vi "Dequeue Events.vi"(8 "error in (no error)":errorcluster, 10 "timeout in ms (-1)":i32, 11 "Queue in":refnum<queue>) -> (0 "error out":errorcluster, 2 "timed out?":bool, 3 "Actor Events":T1)   [LabVIEW 2017, in "Command Handler.lvlib" / "Command Handler.lvclass"]
uses:
  Command Handler.lvclass
  Type Defs/Event Cluster.ctl
  Command Parent/Command.lvclass
  Type Defs/Command Handler Data.ctl
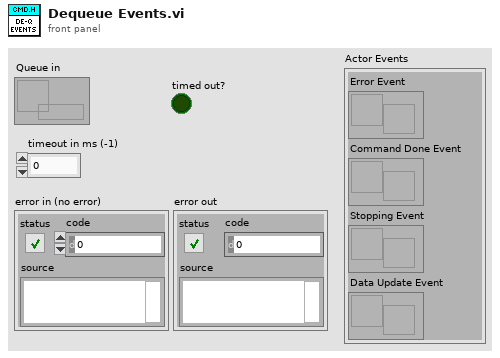
[diagram p1: front panel]
types:
  T1 = typedef "Command Handler.lvlib/Command Handler.lvclass/Event Cluster.ctl" = cluster{"Error Event":refnum<user-event>, "Command Done Event":refnum<user-event>, "Stopping Event":refnum<user-event>, "Data Update Event":refnum<user-event>}
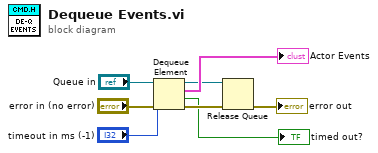
[diagram p0: block diagram]
diagram:
  n1 = Dequeue Element(queue="Queue in", timeout in ms (-1)="timeout in ms (-1)", error in (no error)="error in (no error)") -> (queue out=w6:refnum<queue>, element=→"Actor Events":T1, timed out?=→"timed out?":bool, error out=w5:errorcluster)
  n2 = Release Queue(queue=w6, error in (no error)=w5) -> (error out=→"error out":errorcluster)  [unwired: 1 in, 2 out]
